vi "Curtin_PlaySound.vi"(8 "Task":enum16{"play", "save"}(ring), 10 "all waveforms":waveform(dbl)[](array[waveform]), 11 "device ID":u32) -> (0 "error out":errorcluster)   [LabVIEW 2022 SP3]
uses:
  <vilib>/sound2/lvsound2.llb/Sound Output Write Simple (DBL2).vi
panel:
  in  "Timeout (sec)":dbl=-1.0
  in  "Resolution (bits)":i32=16
  out "Waveform Graph":waveform(dbl)[](graph)
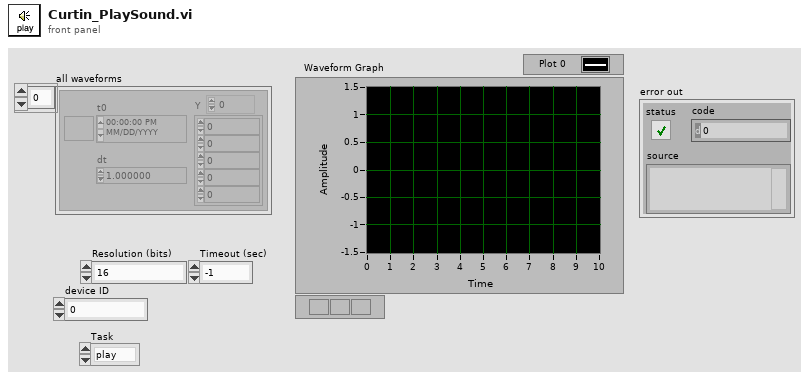
[diagram p1: front panel]
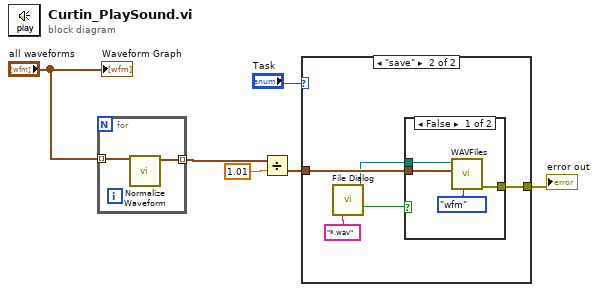
[diagram p0: block diagram]
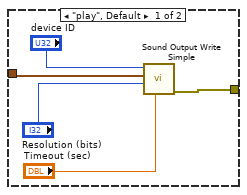
[diagram p2: hidden frame]
diagram:
  n1 = for {
    tunnel: "all waveforms" -> [w8] mode=indexing
    tunnel: [w7] -> w4 mode=indexing
    n2 = call <vilib>:"Normalize Waveform.vi"("waveform in"=w8) -> ("normalized waveform"=w7:waveform(dbl))  [unwired: 7 in, 3 out]
  }
  n3 = Divide(x=w4, y=1.01 ("scale")) -> (x/y=w5:waveform(dbl)[])
  n4 = case shown="\"save\"" "Task" {
    tunnel: w5 -> [w13 w18]
    tunnel: [w12 w17] -> w1
    frame "play", Default {
      n5 = call-poly <vilib>:"Sound Output Write Simple.vi"("timeout (sec)"="Timeout (sec)", "bits per sample"="Resolution (bits)", "data"=w13, "device ID"="device ID") -> ("error out"=w12:errorcluster)  [unwired: 7 in]
    }
    frame "save" {
      n6 = call "File Dialog"("pattern (all files)"="*.wav" ("pattern label")) -> ("selected path"=w15:path, "cancelled"=w14:bool)  [unwired: 11 in, 2 out]
      n7 = case shown="False" w14 {
        tunnel: w18 -> [w21 _]
        tunnel: [w20 _] -> w17
        tunnel: w15 -> [w19 _]
        frame False {
          n8 = call "WAVFiles.vi"("Task"=enum16{"Read", "Write", "wfm"}."wfm", "Wfm data"=w21, "WAV File"=w19) -> ("error out"=w20:errorcluster)  [unwired: 5 in, 3 out]
        }
        frame True {
        }
      }
    }
  }
  "error out" <- w1
  "Waveform Graph" <- "all waveforms"
